vi "create.from_cluster_pairs.vi"(8 "error in":errorcluster, 10 "properties":cluster{"name":string, "value":string}[](array[cluster])) -> (0 "error out":errorcluster, 3 "properties out":refnum<class "properties.lvclass">)   [LabVIEW 2020, in "nominal types.lvlib" / "properties.lvclass"]
uses:
  properties.lvclass
  properties.lvclass/properties.ctl
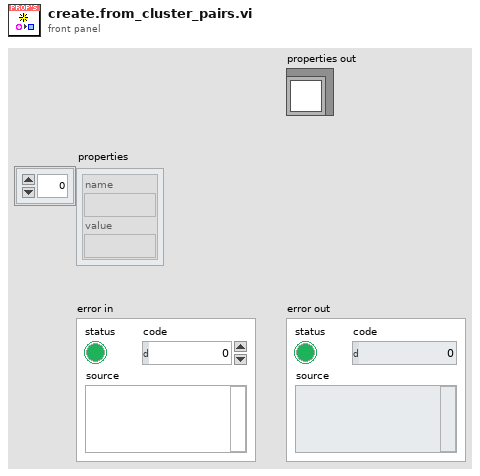
[diagram p1: front panel]
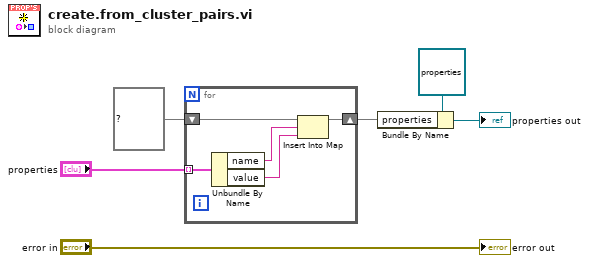
[diagram p0: block diagram]
diagram:
  n1 = for {
    shift-right: [w7] -> w2
    shift-left: map{string, string} {} ("properties") -> [w10]
    tunnel: "properties" -> [w11] mode=indexing
    n2 = Unbundle By Name(w11) -> ("name"=w9:string, "value"=w8:string)
    n3 = Insert Into Map(map in=w10, key=w9, value=w8) -> (map out=w7:map{string, string})  [unwired: 2 out]
  }
  n4 = Bundle By Name(cluster=refnum<class "properties.lvclass"> refnum ("properties out"), "properties"=w2) -> (→"properties out":refnum<class "properties.lvclass">)
  "error out" <- "error in"
